vi "SD_Gen_Random_Frame.vi"(8 "error in (no error)":errorcluster) -> (0 "error out":errorcluster, 3 "Generated data":T1 {"Measurements and statistics"."Running, perc. of time" format="%05.2f"})   [LabVIEW 2018, in "Stream Data.lvlib"]
uses:
  Stream Data.lvlib
  SubVi's/Controls/CTL_Full_data_frame.ctl
  SubVi's/Controls/CTL_Animal_Coordinates_and_Speed.ctl
  SubVi's/Controls/CTL_Measurements_and_Statistics.ctl
  Send Frame Argument--cluster.ctl
  <userlib>/_OpenG.lib/numeric/numeric.llb/Random Number Within Range - DBL__ogtk.vi
  Common_Resources.lvlib
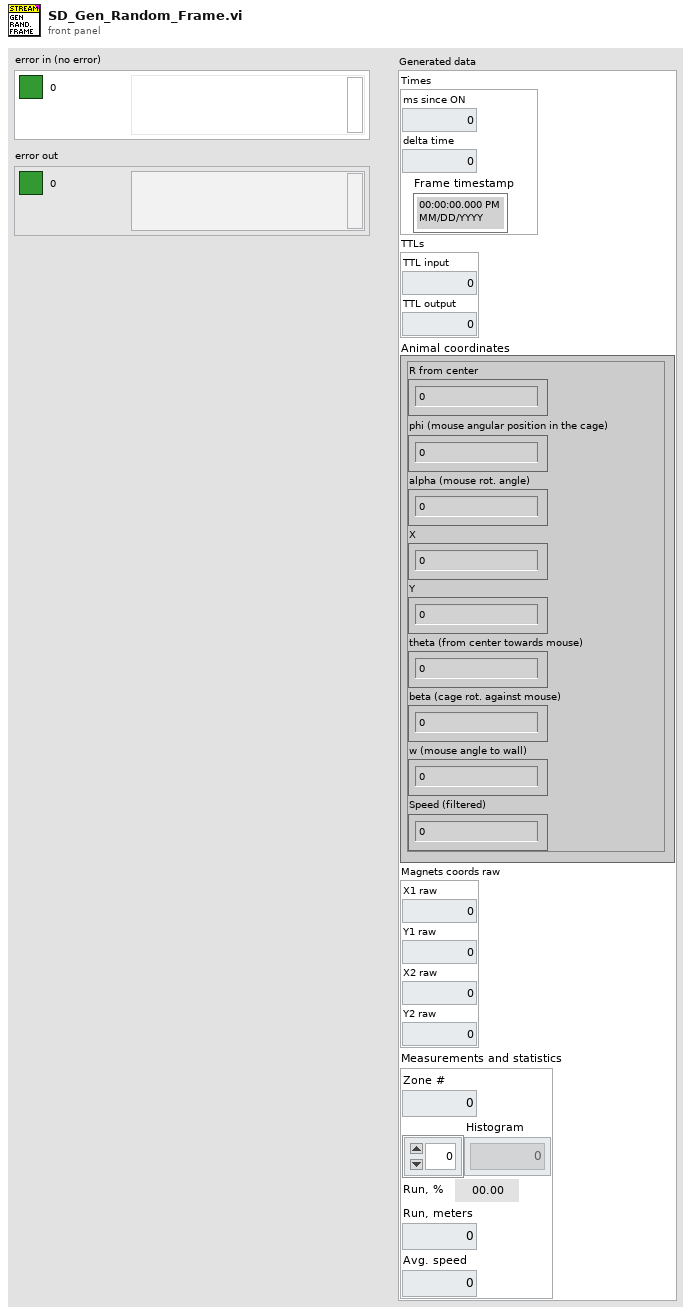
[diagram p1: front panel]
types:
  T1 = typedef "Common_Resources.lvlib/CTL_Full_data_frame.ctl" = cluster{"Times":cluster{"ms since ON":u32, "delta time":u32, "Frame timestamp":timestamp}, "TTLs":cluster{"TTL input":i16, "TTL output":i16}, "Animal coordinates":T2, "Magnets coords raw":cluster{"X1 raw":dbl, "Y1 raw":dbl, "X2 raw":dbl, "Y2 raw":dbl}, "Measurements and statistics":T3}
  T2 = typedef "Common_Resources.lvlib/CTL_Animal_Coordinates_and_Speed.ctl" = cluster{"R from center":dbl, "phi (mouse angular position in the cage)":dbl, "alpha (mouse rot. angle)":dbl, "X":dbl, "Y":dbl, "theta (from center towards mouse)":dbl, "beta (cage rot. against mouse)":dbl, "w (mouse angle to wall)":dbl, "Speed (filtered)":dbl}
  T3 = typedef "Common_Resources.lvlib/CTL_Measurements_and_Statistics.ctl" = cluster{"Zone #":i8, "Histogram":dbl[], "Running, perc. of time":dbl, "Run, meters":dbl, "Avg. speed":dbl}
  T4 = typedef "Stream Data.lvlib/Send Frame Argument--cluster.ctl" = cluster{"Data in":T1}
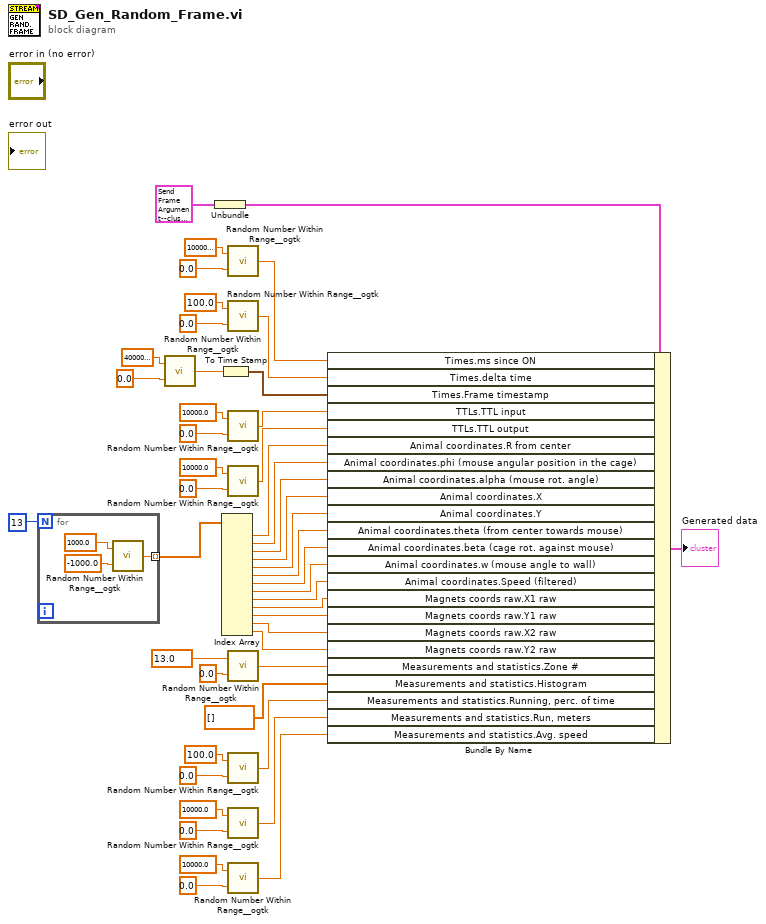
[diagram p0: block diagram]
diagram:
  n1 = for {
    N: 13 -> [_]
    tunnel: [w48] -> w14 mode=indexing
    n2 = call-poly <userlib>:"Random Number Within Range__ogtk.vi"("High"=1000.0, "Low"=-1000.0) -> ("Random Number"=w48:dbl)  [unwired: 3 in]
  }
  n3 = call-poly <userlib>:"Random Number Within Range__ogtk.vi"("High"=4000000000.0, "Low"=0.0) -> ("Random Number"=w36:dbl)  [unwired: 3 in]
  n4 = Unbundle(T4 {"Data in"={"Times"={"ms since ON"=0, "delta time"=0, "Frame timestamp"=timestamp(0 s since 1904-01-01)}, "TTLs"={"TTL input"=0, "TTL output"=0}, "Animal coordinates"={"R from center"=0.0, "phi (mouse angular position in the cage)"=0.0, "alpha (mouse rot. angle)"=0.0, "X"=0.0, "Y"=0.0, "theta (from center towards mouse)"=0.0, "beta (cage rot. against mouse)"=0.0, "w (mouse angle to wall)"=0.0, "Speed (filtered)"=0.0}, "Magnets coords raw"={"X1 raw"=0.0, "Y1 raw"=0.0, "X2 raw"=0.0, "Y2 raw"=0.0}, "Measurements and statistics"={"Zone #"=0, "Histogram"=[], "Running, perc. of time"=0.0, "Run, meters"=0.0, "Avg. speed"=0.0}}} ("Send Frame Argument")) -> ("Data in"=w47:T1)
  n5 = To Time Stamp(1:w36) -> (0:w35:timestamp)
  n6 = Index Array(array=w14) -> (element #1=w13:dbl, element #2=w12:dbl, element #3=w11:dbl, element #4=w10:dbl, element #5=w9:dbl, element #6=w8:dbl, element #7=w7:dbl, element #8=w6:dbl, element #9=w5:dbl, element #10=w4:dbl, element #11=w3:dbl, element #12=w2:dbl, element #13=w1:dbl)  [unwired: 13 in]
  n7 = call-poly <userlib>:"Random Number Within Range__ogtk.vi"("High"=1000000000.0, "Low"=0.0) -> ("Random Number"=w42:dbl)  [unwired: 3 in]
  n8 = call-poly <userlib>:"Random Number Within Range__ogtk.vi"("High"=100.0, "Low"=0.0) -> ("Random Number"=w39:dbl)  [unwired: 3 in]
  n9 = call-poly <userlib>:"Random Number Within Range__ogtk.vi"("High"=10000.0, "Low"=0.0) -> ("Random Number"=w32:dbl)  [unwired: 3 in]
  n10 = call-poly <userlib>:"Random Number Within Range__ogtk.vi"("High"=10000.0, "Low"=0.0) -> ("Random Number"=w29:dbl)  [unwired: 3 in]
  n11 = call-poly <userlib>:"Random Number Within Range__ogtk.vi"("High"=13.0, "Low"=0.0) -> ("Random Number"=w27:dbl)  [unwired: 3 in]
  n12 = call-poly <userlib>:"Random Number Within Range__ogtk.vi"("High"=100.0, "Low"=0.0) -> ("Random Number"=w23:dbl)  [unwired: 3 in]
  n13 = call-poly <userlib>:"Random Number Within Range__ogtk.vi"("High"=10000.0, "Low"=0.0) -> ("Random Number"=w20:dbl)  [unwired: 3 in]
  n14 = call-poly <userlib>:"Random Number Within Range__ogtk.vi"("High"=10000.0, "Low"=0.0) -> ("Random Number"=w17:dbl)  [unwired: 3 in]
  n15 = Bundle By Name(cluster=w47, "Times.ms since ON"=w42, "Times.delta time"=w39, "Times.Frame timestamp"=w35, "TTLs.TTL input"=w32, "TTLs.TTL output"=w29, "Animal coordinates.R from center"=w13, "Animal coordinates.phi (mouse angular position in the cage)"=w12, "Animal coordinates.alpha (mouse rot. angle)"=w11, "Animal coordinates.X"=w10, "Animal coordinates.Y"=w9, "Animal coordinates.theta (from center towards mouse)"=w8, "Animal coordinates.beta (cage rot. against mouse)"=w7, "Animal coordinates.w (mouse angle to wall)"=w6, "Animal coordinates.Speed (filtered)"=w5, "Magnets coords raw.X1 raw"=w4, "Magnets coords raw.Y1 raw"=w3, "Magnets coords raw.X2 raw"=w2, "Magnets coords raw.Y2 raw"=w1, "Measurements and statistics.Zone #"=w27, "Measurements and statistics.Histogram"=dbl[] [], "Measurements and statistics.Running, perc. of time"=w23, "Measurements and statistics.Run, meters"=w20, "Measurements and statistics.Avg. speed"=w17) -> (→"Generated data":T1)
